vi "Solenoid Global.vi"() -> ()   [LabVIEW 2015]
uses:
  Solenoid Type Def.ctl
  <vilib>/Rock Robotics/WPI/Solenoid/WPI_SolenoidChannel.ctl
panel:
  in  "Solenoids":T1[](array[typedef])
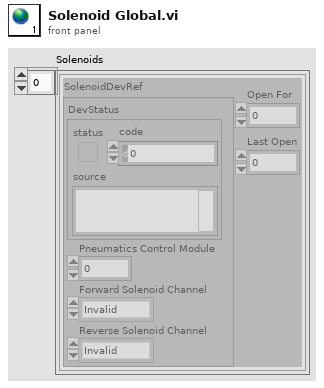
[diagram p1: front panel]
types:
  T1 = typedef "Solenoid Type Def.ctl" = cluster{"SolenoidDevRef":cluster{"DevStatus":errorcluster, "Pneumatics Control Module":u8, "Forward Solenoid Channel":T2, "Reverse Solenoid Channel":T2}, "Open For":dbl, "Last Open":dbl}
  T2 = typedef "WPI_SolenoidChannel.ctl" = enum8{"Solenoid 0", "Solenoid 1", "Solenoid 2", "Solenoid 3", "Solenoid 4", "Solenoid 5", "Solenoid 6", "Solenoid 7", "Invalid"}
diagram:
